vi "sftp_symlink.vi"() -> ()   [LabVIEW 2013]
doc: "Illustrates how to work with symbolic links using SFTP."
uses:
  libssh2/libssh2_init_default.vi
  libssh2/libssh2_session_handshake_tcp.vi
  libssh2/libssh2.lvlib
panel:
  out "realpath":string
  out "readlink":string
  in  "target":string="/"
  in  "path":string="/"
  out "error out":errorcluster
  in  "password":string
  in  "username":string
  in  "hostname":string
  # "Note: This does not work if the symlink already exists."
  # "This is the remote file system object to create a symlink for."
  # "This is the remote file system object to link to (the symlink)."
  # "This is the target of the symlink."
  # "This is the real path of the symlink."
  # "Note: When a symbolic link refers to a symbolic link, then the real path will resolve the path to the effective target."
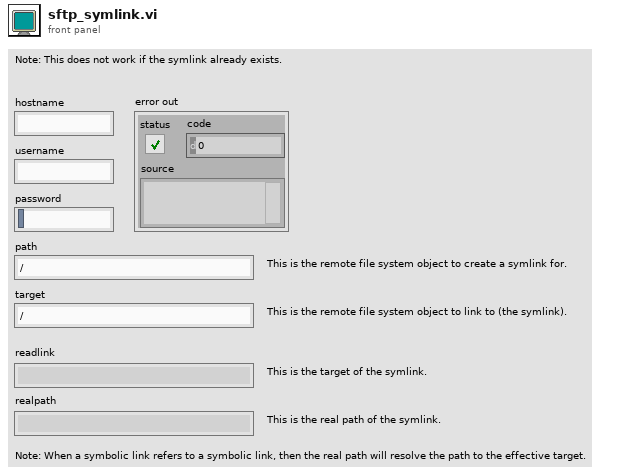
[diagram p1: front panel]
types:
  T1 = typedef "libssh2.lvlib/Session Refnum.ctl" = refnum<k1>
  T2 = typedef "libssh2.lvlib/SFTP Refnum.ctl" = refnum<k1>
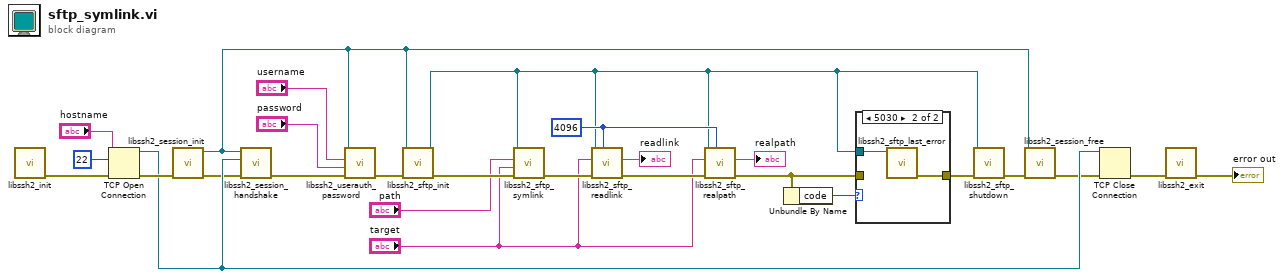
[diagram p0: block diagram]
diagram:
  w3 = u32 4096 ("target_len")
  n1 = call-poly "libssh2_init.vi"() -> ("error out"=w26:errorcluster)  [unwired: 11 in]
  n2 = TCP Open Connection(address="hostname", remote port or service name=u16 22, error in (no error)=w26) -> (connection ID=w24:refnum<k5>, error out=w25:errorcluster)  [unwired: 2 in]
  n3 = call "libssh2_session_init.vi"("error in (no error)"=w25) -> ("error out"=w23:errorcluster, "session"=w16:T1)  [unwired: 9 in]
  n4 = call-poly "libssh2_session_handshake.vi"("error in (no error)"=w23, "tcp connection"=w24, "session"=w16) -> ("error out"=w27:errorcluster)  [unwired: 8 in]
  n5 = call "libssh2_userauth_password.vi"("error in (no error)"=w27, "password"="password", "username"="username", "session"=w16) -> ("error out"=w20:errorcluster)  [unwired: 7 in]
  n6 = call "libssh2_sftp_init.vi"("error in (no error)"=w20, "session"=w16) -> ("error out"=w12:errorcluster, "sftp"=w1:T2)  [unwired: 8 in]
  n7 = call "libssh2_sftp_symlink.vi"("error in (no error)"=w12, "target"="target", "path"="path", "sftp"=w1) -> ("error out"=w8:errorcluster)  [unwired: 7 in]
  n8 = call "libssh2_sftp_readlink.vi"("target_len"=w3, "error in (no error)"=w8, "path"="target", "sftp"=w1) -> ("error out"=w7:errorcluster, "target"=→"readlink":string)  [unwired: 6 in]
  n9 = call "libssh2_sftp_realpath.vi"("maxlen"=w3, "error in (no error)"=w7, "path"="target", "sftp"=w1) -> ("error out"=w5:errorcluster, "target"=→"realpath":string)  [unwired: 6 in]
  n10 = Unbundle By Name(w5) -> ("code"=w9:i32)
  n11 = case shown="5030" w9 {
    tunnel: w5 -> [w28 _]
    tunnel: [w28 w30] -> w10
    tunnel: w1 -> [_ w29]
    frame Default {
    }
    frame 5030 {
      n12 = call "libssh2_sftp_last_error.vi"("sftp"=w29) -> ("error out"=w30:errorcluster)  [unwired: 10 in]
    }
  }
  n13 = call "libssh2_sftp_shutdown.vi"("error in (no error)"=w10, "sftp"=w1) -> ("error out"=w13:errorcluster)  [unwired: 9 in]
  n14 = call "libssh2_session_free.vi"("error in (no error)"=w13, "session"=w16) -> ("error out"=w15:errorcluster)  [unwired: 9 in]
  n15 = TCP Close Connection(connection ID=w24, error in (no error)=w15) -> (error out=w14:errorcluster)  [unwired: 1 in, 1 out]
  n16 = call "libssh2_exit.vi"("error in (no error)"=w14) -> ("error out"=→"error out":errorcluster)  [unwired: 10 in]
